vi "bt_test2.vi"() -> ()   [LabVIEW 2025]
panel:
  in  "Send Button":bool
  in  "TX Message":string
  in  "VI Path":string
  out "String":string
  out "BT Status":bool
  in  "BT Switch":bool
  out "error out":errorcluster
  in  "TX_CHAR_UUID":string
  in  "SERVICE UUID":string
  in  "RX_CHAR_UUID":string
  in  "stop":bool
  in  "Python Script Path":path
  in  "Python Interpreter Path":path
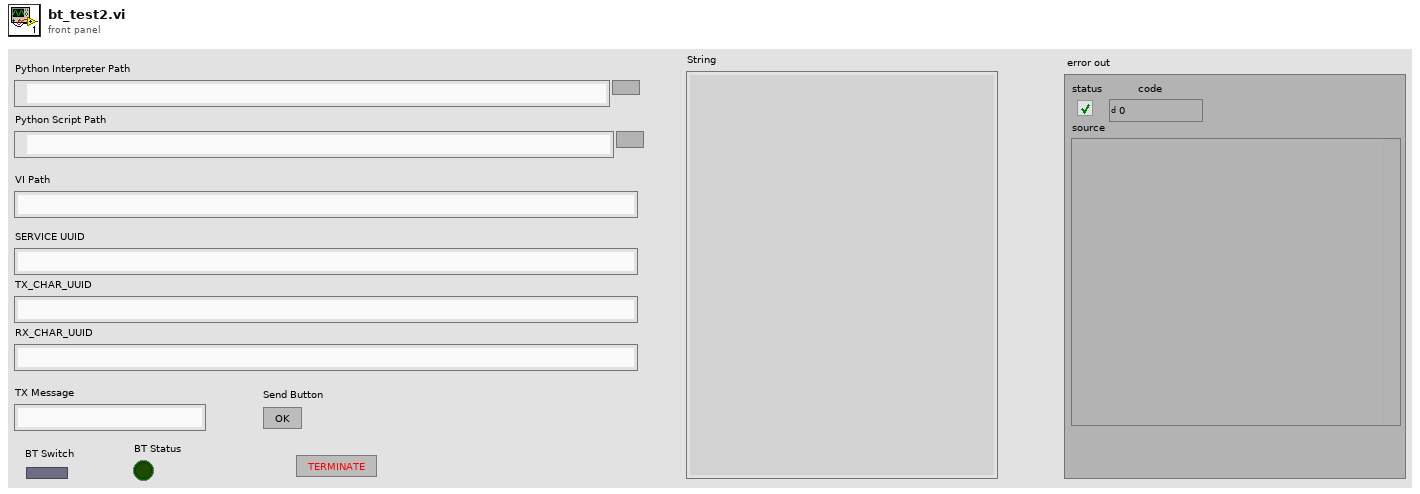
[diagram p1: front panel]
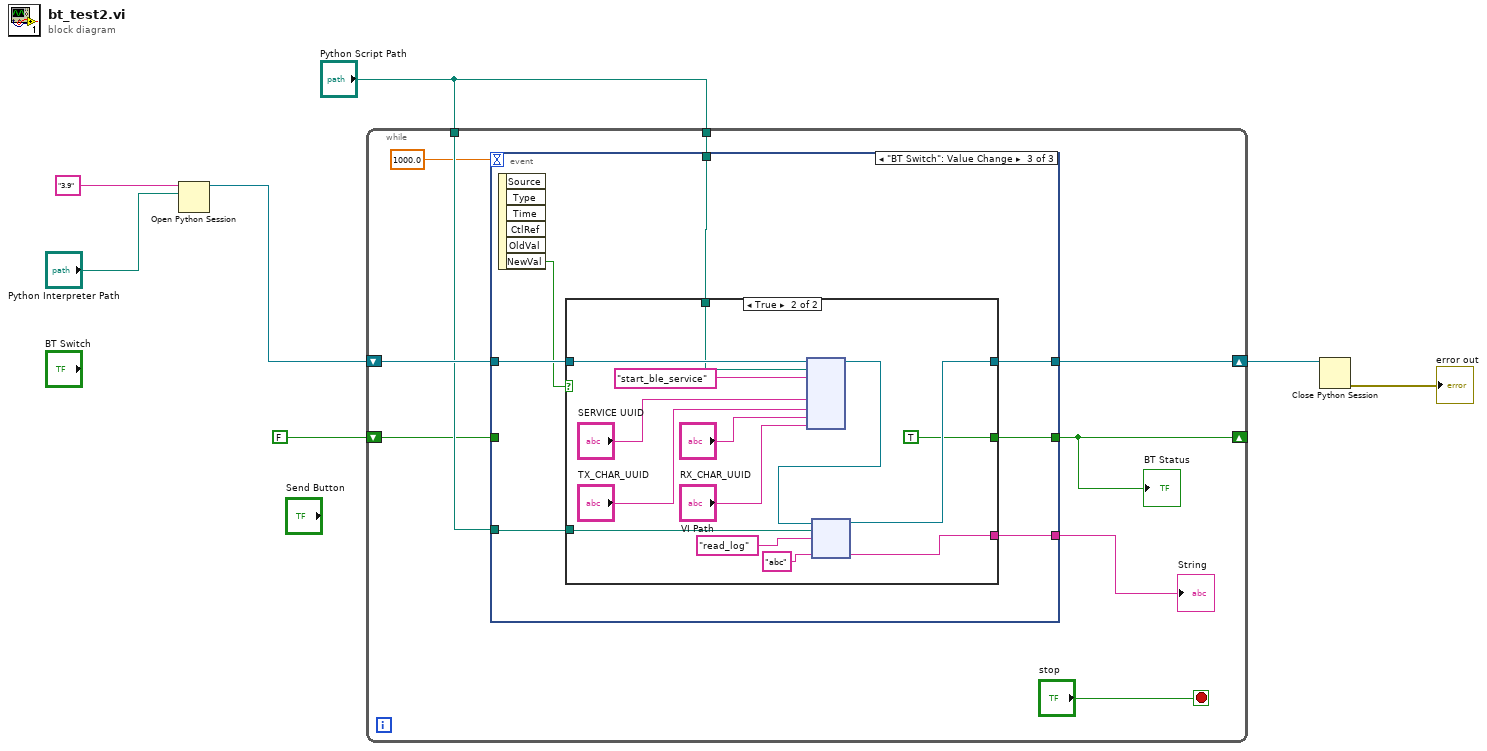
[diagram p0: block diagram]
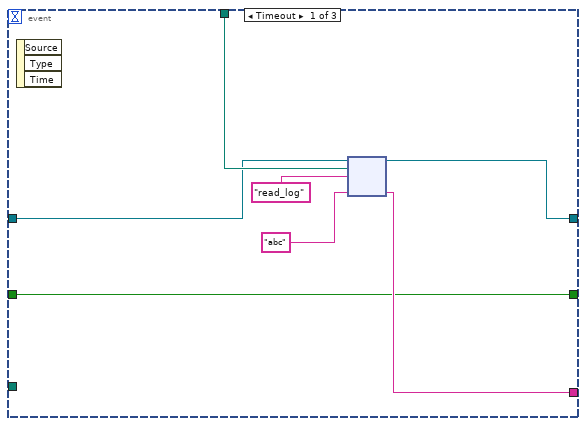
[diagram p2: hidden frame]
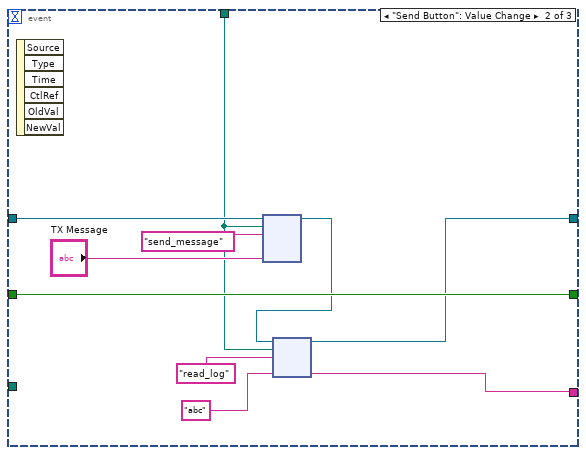
[diagram p3: hidden frame]
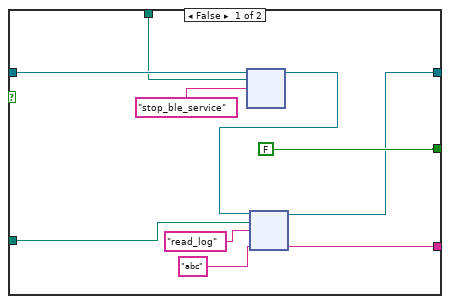
[diagram p4: hidden frame]
diagram:
  n1 = Open Python Session(python version="3.9", python path="Python Interpreter Path") -> (session out=w5:refnum<k35>)  [unwired: 1 in, 1 out]
  n2 = while {
    shift-right: [w12] -> w2
    shift-left: w5 -> [w15]
    shift-right: [w8] -> _
    shift-left: FALSE -> [w9]
    tunnel: "Python Script Path" -> [w14]
    tunnel: "Python Script Path" -> [w13]
    stop <- "stop" stop-if-true
    n3 = event shown="[2] \"BT Switch\": Value Change" {
      selector: _ -> [_ _ _]
      dyn-events: _ -> [_ _ _]
      timeout: 1000.0 -> [_ _ _]
      tunnel: w15 -> [w21 w31 w40]
      tunnel: [w20 w25 w39] -> w12
      tunnel: w14 -> [w22 w24 w38]
      tunnel: w13 -> [_ _ w37]
      tunnel: [w18 w27 w36] -> w11
      tunnel: w9 -> [w17 w30 _]
      tunnel: [w17 w30 w34] -> w8
      event Timeout {
        n4 = event-data() -> ()  [unwired: 1 in, 3 out]
        n5 = node(w21, w22, "read_log", "abc") -> (w20:refnum<k35>, w18:string)  [unwired: 1 in, 3 out]
      }
      event "Send Button": Value Change {
        n6 = event-data() -> ()  [unwired: 1 in, 6 out]
        n7 = node(w31, w24, "send_message", "TX Message") -> (w26:refnum<k35>)  [unwired: 4 in, 3 out]
        n8 = node(w26, w24, "read_log", "abc") -> (w25:refnum<k35>, w27:string)  [unwired: 1 in, 3 out]
      }
      event "BT Switch": Value Change {
        n9 = event-data() -> ("NewVal"=w35:bool)  [unwired: 1 in, 5 out]
        n10 = case shown="True" w35 {
          tunnel: w40 -> [w49 w63]
          tunnel: [w45 w60] -> w39
          tunnel: [FALSE TRUE] -> w34
          tunnel: w38 -> [w43 w59]
          tunnel: w37 -> [w44 w58]
          tunnel: [w41 w55] -> w36
          frame False {
            n11 = node(w49, w43, "stop_ble_service") -> (w46:refnum<k35>)  [unwired: 3 in, 3 out]
            n12 = node(w46, w44, "read_log", "abc") -> (w45:refnum<k35>, w41:string)  [unwired: 1 in, 3 out]
          }
          frame True {
            n13 = node(w63, w59, "start_ble_service", "SERVICE UUID", "TX_CHAR_UUID", "RX_CHAR_UUID", "VI Path") -> (w61:refnum<k35>)  [unwired: 7 in, 3 out]
            n14 = node(w61, w58, "read_log", "abc") -> (w60:refnum<k35>, w55:string)  [unwired: 1 in, 3 out]
          }
        }
      }
    }
    "BT Status" <- w8
    "String" <- w11
  }
  n15 = Close Python Session(session in=w2) -> (11:→"error out":errorcluster)  [unwired: 1 in]
